vi "Initialize1.vi"(6 "Files in":T1, 8 "Status/Errors in":refnum<vi>, 9 "Control Parameters [] in":T2[](array[typedef]) {"Aux Byte Value" format="%02x"; "Max Real Value" format="%#_6e"; "Min Real Value" format="%#_6e"; "dReal/dByte" format="%#_6e"; "Byte Value" format="%02x"; "Identifier" format="%02x"}, 10 "Mode in":T5={"Mode"=enum."Dialog", "Expert?"=FALSE, "Dialog?"=FALSE}) -> (0 "Status/Errors out":refnum<vi>, 1 "Control Parameters [] out":T2[](array[typedef]) {"Aux Byte Value" format="%02x"; "Max Real Value" format="%#_6e"; "Min Real Value" format="%#_6e"; "dReal/dByte" format="%#_6e"; "Byte Value" format="%02x"; "Identifier" format="%02x"}, 2 "Mode out":T5={"Mode"=enum."Dialog", "Expert?"=FALSE, "Dialog?"=FALSE}, 4 "Files out":T1, 5 "Mode":T4(ring))   [LabVIEW 2013]
uses:
  Controls/Mode.ctl
  Controls/Control_Parameters.ctl
  Controls/Master.ctl
  Controls/Files.ctl
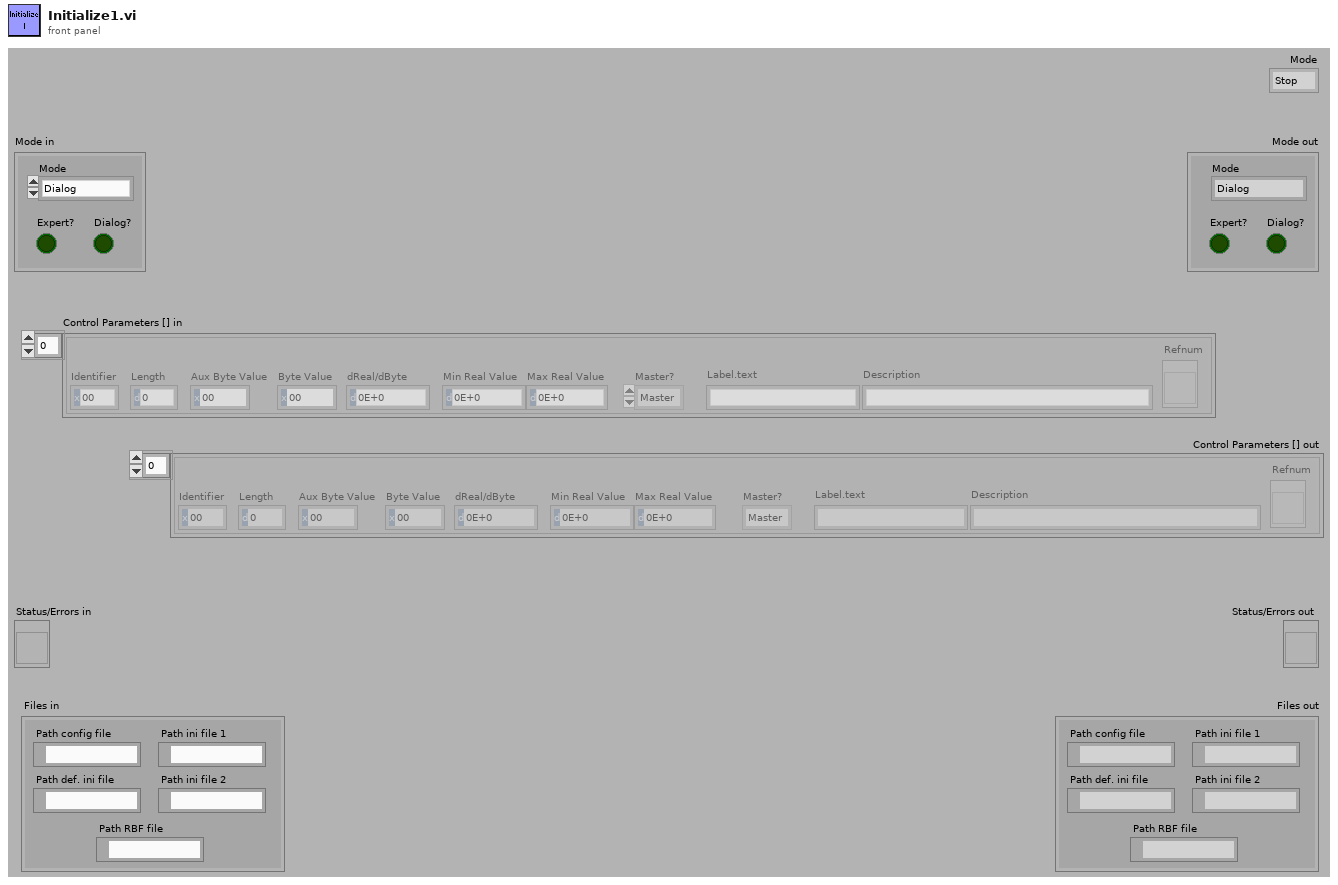
[diagram p1: front panel]
types:
  T1 = typedef "Files.ctl" = cluster{"Path config file":path, "Path def. ini file":path, "Path ini file 1":path, "Path ini file 2":path, "Path RBF file":path}
  T2 = typedef "Control_Parameters.ctl" = cluster{"Identifier":u8, "Length":u16, "Byte Value":u32, "dReal/dByte":dbl, "Min Real Value":dbl, "Max Real Value":dbl, "Master?":T3, "Label.text":string, "Description":string, "Refnum":refnum<vi>, "Aux Byte Value":u32}
  T3 = typedef "Master.ctl" = enum16{"Master", "Slave", "General"}
  T4 = enum8{"Stop", "Dialog", "Hisparc II", "Hisparc II DAQ", "Alignment"}
  T5 = typedef "Mode.ctl" = cluster{"Mode":enum8{"Stop", "Dialog", "Hisparc II", "Hisparc II DAQ", "Alignment"}, "Expert?":bool, "Dialog?":bool}
  T6 = typedef "Configuration_File_Parameters.ctl" = cluster{"Mode":T5, "Hardware":enum8{"None", "HiSPARC I", "HiSPARC II", "HiSPARC III"}, "Time difference":string}
  T7 = enum8{"None", "HiSPARC I", "HiSPARC II", "HiSPARC III"}
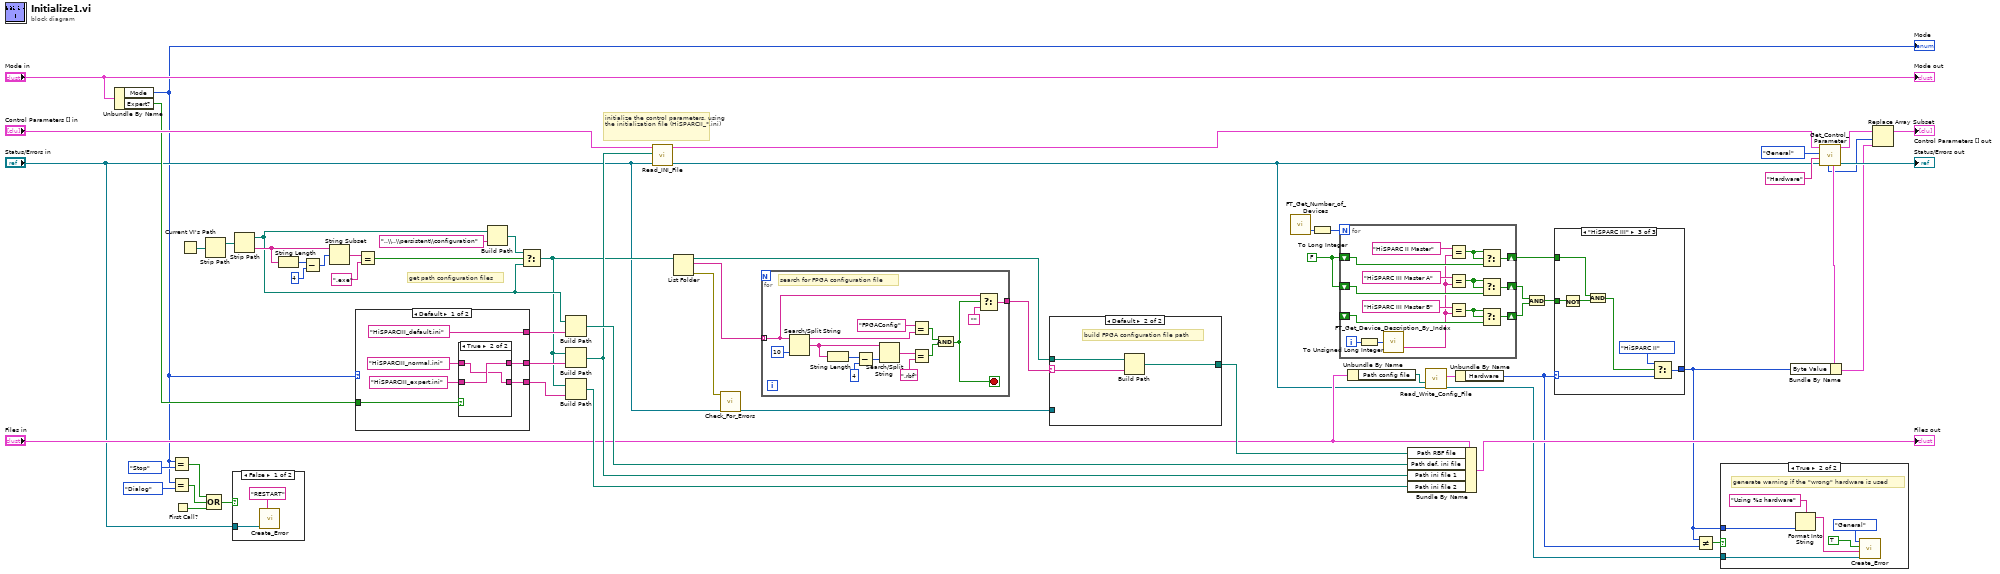
[diagram p0: block diagram]
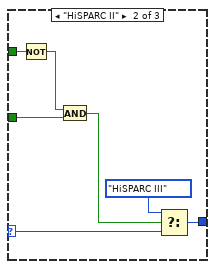
[diagram p5: hidden frame]
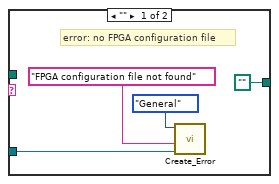
[diagram p6: hidden frame]
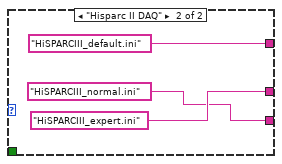
[diagram p8: hidden frame]
diagram:
  w20 = FALSE
  # "get path configuration files"
  # "initialize the control parameters, using\nthe initialization file (HiSPARCII_*.ini)"
  n1 = Unbundle By Name("Mode in") -> ("Mode"=w1:T4, "Expert?"=w60:bool)
  "Mode" <- w1
  n2 = Equal?(x=w1, y=T4."Stop") -> (x = y?=w2:bool)
  n3 = Equal?(x=w1, y=T4."Dialog") -> (x = y?=w5:bool)
  n4 = First Call?() -> (First Call?: T/F=w6:bool)
  n5 = Current VI's Path() -> (path=w52:path)
  n6 = Strip Path(path=w52) -> (stripped path=w42:path)  [unwired: 1 out]
  n7 = Compound Arithmetic op=OR(w2, w5, w6) -> (w8:bool)
  n8 = case shown="False" w8 {
    tunnel: "Status/Errors in" -> [w63 _]
    frame False {
      n9 = call "Create_Error.vi"("Restart text (\"\")"="RESTART" ("Restart text (\"\")"), "Status/Errors in"=w63) -> ()  [unwired: 4 in, 6 out]
    }
    frame True {
    }
  }
  n10 = Strip Path(path=w42) -> (stripped path=w41:path, name=w48:string)
  n11 = String Length(string=w48) -> (length=w51:i32)
  n12 = Subtract(x=w51, y=4) -> (x-y=w49:i32)
  n13 = String Subset(string=w48, offset (0)=w49) -> (substring=w47:string)  [unwired: 1 out]
  n14 = case shown="Default" w1 {
    tunnel: w60 -> [w68 _]
    tunnel: ["HiSPARCIII_default.ini" "HiSPARCIII_default.ini"] -> w59
    tunnel: [w67 "HiSPARCIII_expert.ini"] -> w58
    tunnel: [w65 "HiSPARCIII_normal.ini"] -> w57
    frame Default {
      n15 = case shown="True" w68 {
        tunnel: [w71 w73] -> w67
        tunnel: "HiSPARCIII_normal.ini" -> [w71 w72]
        tunnel: [w70 w72] -> w65
        tunnel: "HiSPARCIII_expert.ini" -> [w70 w73]
        frame False {
        }
        frame True {
        }
      }
    }
    frame "Hisparc II DAQ" {
    }
  }
  n16 = Equal?(x=w47, y=".exe") -> (x = y?=w45:bool)
  n17 = Build Path(base path=w41, name or relative path="..\\..\\persistent\\configuration") -> (appended path=w43:path)
  n18 = Select(t=w43, s=w45, f=w41) -> (s? t:f=w35:path)
  n19 = Build Path(base path=w41, name or relative path=w59) -> (appended path=w56:path)
  n20 = Build Path(base path=w35, name or relative path=w58) -> (appended path=w54:path)
  n21 = Build Path(base path=w35, name or relative path=w57) -> (appended path=w55:path)
  n22 = call "Read_INI_File.vi"("Status/Errors in"="Status/Errors in", "Path ini file in"=w54, "Control Parameters [] in"="Control Parameters [] in") -> ("Status/Errors out"=w10:refnum<vi>, "Control Parameters [] out"=w11:T2[])  [unwired: 1 in, 6 out]
  n23 = List Folder(path=w35) -> (path out=w38:path, filenames=w39:string[], error out=w40:errorcluster)  [unwired: 1 in, 3 out]
  n24 = call "Check_For_Errors.vi"("Status/Errors in"="Status/Errors in", "error in"=w40) -> ("Status/Errors out"=w37:refnum<vi>)  [unwired: 9 out]
  n25 = for {
    tunnel: w39 -> [w84] mode=indexing
    tunnel: [w82] -> w36
    stop <- w85 stop-if-true
    # "search for FPGA configuration file"
    n26 = Search/Split String(string=w84, offset (0)=10 ("length (rest)")) -> (substring before match=w79:string, match + rest of string=w78:string)  [unwired: 2 out]
    n27 = String Length(string=w78) -> (length=w88:i32)
    n28 = Subtract(x=w88, y=4) -> (x-y=w86:i32)
    n29 = Search/Split String(string=w78, offset (0)=w86) -> (match + rest of string=w90:string)  [unwired: 1 in, 2 out]
    n30 = Equal?(x="FPGAConfig" ("y"), y=w79) -> (x = y?=w77:bool)
    n31 = Equal?(x=w90, y=".rbf") -> (x = y?=w81:bool)
    n32 = And(x=w77, y=w81) -> (x .and. y?=w85:bool)
    n33 = Select(t=w84, s=w85, f="") -> (s? t:f=w82:string)
  }
  n34 = case shown="Default" w36 {
    selector: w36 -> [_ w96]
    tunnel: [path "" w98] -> w34
    tunnel: w38 -> [_ w97]
    tunnel: w37 -> [w93 _]
    frame "" {
      # "error: no FPGA configuration file"
      n35 = call "Create_Error.vi"("Status/Errors in"=w93, "HiSPARC error"="FPGA configuration file not found", "Master?"=Master."General") -> ()  [unwired: 3 in, 6 out]
    }
    frame Default {
      # "build FPGA configuration file path"
      n36 = Build Path(base path=w97, name or relative path=w96) -> (appended path=w98:path)
    }
  }
  n37 = call "FT_Get_Number_of_Devices.vi"() -> ("Number of Devices"=w22:u16)  [unwired: 1 out]
  n38 = To Long Integer(number=w22) -> (32bit integer=w21:i32)
  n39 = for {
    N: w21 -> [_]
    shift-right: [w108] -> w19
    shift-left: w20 -> [w109]
    shift-right: [w104] -> w17
    shift-left: w20 -> [w105]
    shift-right: [w101] -> w18
    shift-left: _ -> [w100]
    i -> [w112]
    n40 = To Unsigned Long Integer(number=w112) -> (unsigned 32bit integer=w113:u32)
    n41 = call "FT_Get_Device_Description_By_Index.vi"("Device Index"=w113) -> ("Device Description"=w99:string)  [unwired: 1 out]
    n42 = Equal?(x="HiSPARC II Master", y=w99) -> (x = y?=w110:bool)
    n43 = Equal?(x="HiSPARC III Master A", y=w99) -> (x = y?=w107:bool)
    n44 = Equal?(x="HiSPARC III Master B", y=w99) -> (x = y?=w102:bool)
    n45 = Select(t=w110, s=w110, f=w109) -> (s? t:f=w108:bool)
    n46 = Select(t=w107, s=w107, f=w105) -> (s? t:f=w104:bool)
    n47 = Select(t=w102, s=w102, f=w100) -> (s? t:f=w101:bool)
  }
  n48 = Unbundle By Name("Files in") -> ("Path config file"=w24:path)
  n49 = Bundle By Name(cluster="Files in", "Path RBF file"=w34, "Path def. ini file"=w56, "Path ini file 1"=w54, "Path ini file 2"=w55) -> (→"Files out":T1)
  n50 = call "Read_Write_Config_File.vi"("Status/Errors in"=w10, "Path config file in"=w24) -> ("Status/Errors out"=w12:refnum<vi>, "Parameters out"=w26:T6)  [unwired: 2 in, 6 out]
  n51 = Unbundle By Name(w26) -> ("Hardware"=w14:T7)
  n52 = And(x=w17, y=w18) -> (x .and. y?=w16:bool)
  n53 = case shown="\"HiSPARC III\"" w14 {
    selector: w14 -> [w114 w117 w126]
    tunnel: w19 -> [_ w121 w123]
    tunnel: w16 -> [_ w119 w128]
    tunnel: [w114 w116 w125] -> w13
    frame Default {
    }
    frame "HiSPARC II" {
      n54 = Not(x=w121) -> (.not. x?=w120:bool)
      n55 = And(x=w120, y=w119) -> (x .and. y?=w118:bool)
      n56 = Select(t=T7."HiSPARC III", s=w118, f=w117) -> (s? t:f=w116:T7)
    }
    frame "HiSPARC III" {
      n57 = Not(x=w128) -> (.not. x?=w122:bool)
      n58 = And(x=w123, y=w122) -> (x .and. y?=w127:bool)
      n59 = Select(t=T7."HiSPARC II", s=w127, f=w126) -> (s? t:f=w125:T7)
    }
  }
  n60 = Not Equal?(x=w13, y=w14) -> (x != y?=w15:bool)
  n61 = case shown="True" w15 {
    tunnel: w13 -> [_ w133]
    tunnel: w12 -> [_ w129]
    frame False {
    }
    frame True {
      # "generate warning if the \"wrong\" hardware is used"
      n62 = Format Into String(format string="Using %s hardware" ("HiSPARC error"), w133) -> (resulting string=w131:string)  [unwired: 2 in, 1 out]
      n63 = call "Create_Error.vi"("Status/Errors in"=w129, "HiSPARC error"=w131, "Warning? (false)"=TRUE, "Master?"=Master."General") -> ()  [unwired: 2 in, 6 out]
    }
  }
  n64 = call "Get_Control_Parameter.vi"("Status/Errors in"=w10, "Label.text in"="Hardware", "Master?"=Master."General", "Control Parameters [] in"=w11) -> ("Status/Errors out"=→"Status/Errors out":refnum<vi>, "Control Parameters [] out"=w32:T2[], "Control Parameter"=w28:T2, "index"=w23:i32)  [unwired: 4 out]
  n65 = Bundle By Name(cluster=w28, "Byte Value"=w13) -> (w27:T2)
  n66 = Replace Array Subset(array=w32, new element=w27, index=w23) -> (→"Control Parameters [] out":T2[])
  "Mode out" <- "Mode in"
